vi "parse_save_gear_to_batch_response.vi"(7 "gear_ok?":i32, 8 "error_in":errorcluster, 10 "SQL_result":variant, 11 "current_batch_count":u16) -> (0 "error_out":errorcluster, 3 "current_batch_count":u16)   [LabVIEW 2019]
uses:
  _misc/AULocalize/SubVIs/Get Localized Phrase Compact Interface 0D.vi
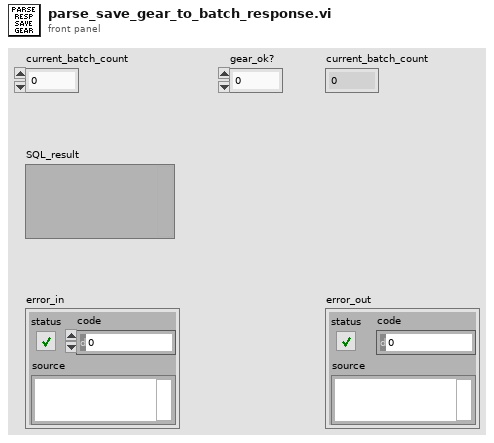
[diagram p1: front panel]
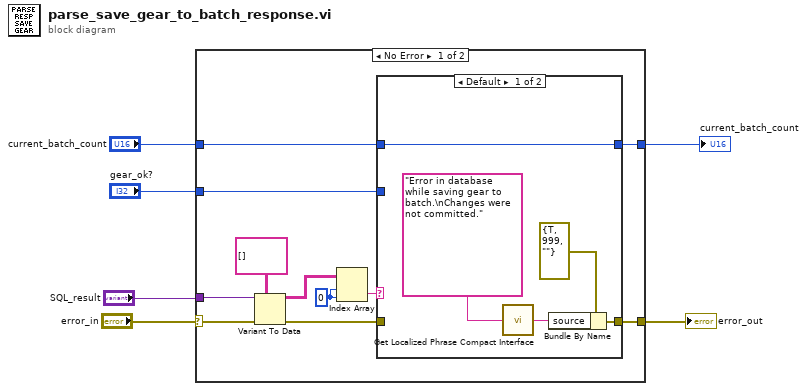
[diagram p0: block diagram]
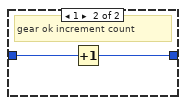
[diagram p3: hidden frame]
diagram:
  n1 = case shown="No Error" "error_in" {
    selector: "error_in" -> [w15 w31]
    tunnel: "SQL_result" -> [w16 _]
    tunnel: [w11 w31] -> w5
    tunnel: "current_batch_count" -> [w9 w30]
    tunnel: [w8 w30] -> w2
    tunnel: "gear_ok?" -> [w7 _]
    frame No Error {
      w10 = 0 ("disabled index (col)")
      n2 = Variant To Data(error in=w15, type=string[][] [], Variant=w16) -> (data=w13:string[][], error out=w12:errorcluster)
      n3 = Index Array(array=w13, index (row)=w10, index (col)=w10) -> (element=w17:string)
      n4 = case shown="Default" w17 {
        tunnel: w12 -> [_ w26]
        tunnel: [w22 w26] -> w11
        tunnel: w9 -> [w19 w25]
        tunnel: [w19 w24] -> w8
        tunnel: w7 -> [_ w23]
        frame Default {
          n5 = call-poly "Get Localized Phrase Compact Interface.vi"("Key"="Error in database while saving gear to batch.\nChanges were not committed." ("source")) -> ("Translated Phrase"=w18:string)
          n6 = Bundle By Name(cluster=errorcluster {"status"=TRUE, "code"=999, "source"=""} ("error out"), "source"=w18) -> (w22:errorcluster)
        }
        frame "1" {
          n7 = case shown="Default" w23 {
            tunnel: w25 -> [w27 w29]
            tunnel: [w27 w28] -> w24
            frame Default {
              # "gear nok, do not increment"
            }
            frame 1 {
              # "gear ok increment count"
              n8 = Increment(x=w29) -> (x+1=w28:u16)
            }
          }
        }
      }
    }
    frame Error {
    }
  }
  "error_out" <- w5
  "current_batch_count" <- w2
